vi "create event registration.vi"(8 "error in":errorcluster, 11 "connection in":refnum<class "connection.lvclass">) -> (0 "error out":errorcluster, 3 "Event Registration Refnum":refnum<event-registration>)   [LabVIEW 2016, in "connection.lvclass"]
uses:
  connection.lvclass
  dllwrapper/tls action complete user event.ctl
  dllwrapper/tls data user event.ctl
  connection.lvclass/connection.ctl
  dllwrapper/async tls dl.lvlib
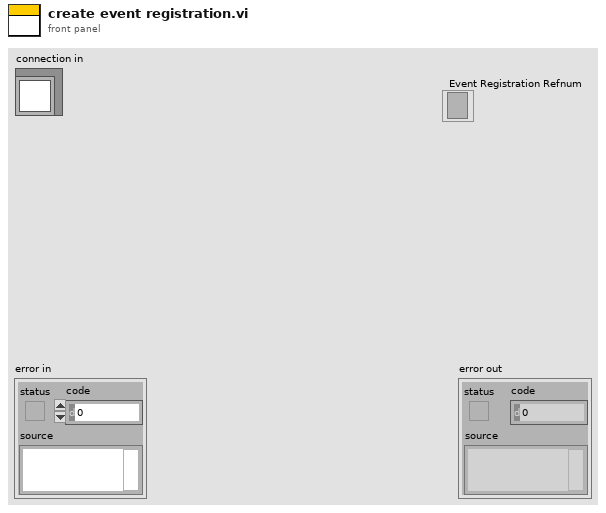
[diagram p1: front panel]
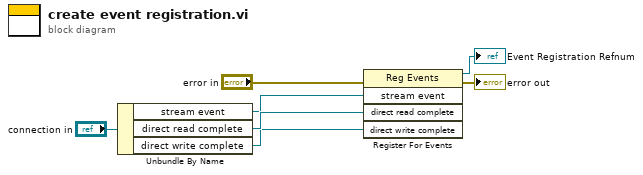
[diagram p0: block diagram]
diagram:
  n1 = Unbundle By Name("connection in") -> ("stream event"=w3:refnum<user-event>, "direct read complete"=w4:refnum<user-event>, "direct write complete"=w2:refnum<user-event>)
  n2 = register-events(error in="error in", w3, w4, w2) -> (reference out=→"Event Registration Refnum":refnum<event-registration>, error out=→"error out":errorcluster)  [unwired: 1 in]
